vi "Trigger Sweep.vi"() -> ()   [LabVIEW 2011]
panel:
  out "Shots Measured":ext[][](array[numeric]) format="%#_10g"
  in  "Channel Delay (milliseconds)":u32=2500
  in  "Shot Delay (miliseconds)":u32
  in  "Shots":i32
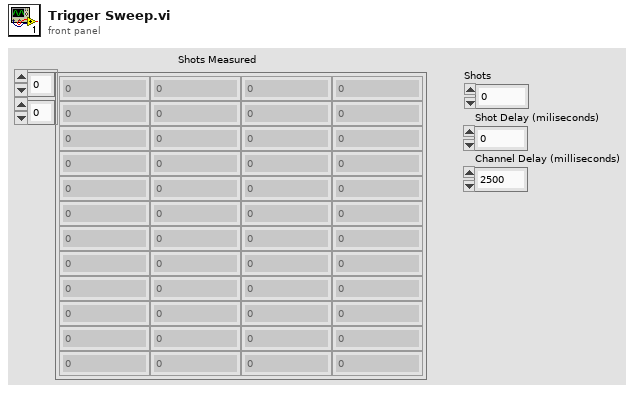
[diagram p1: front panel]
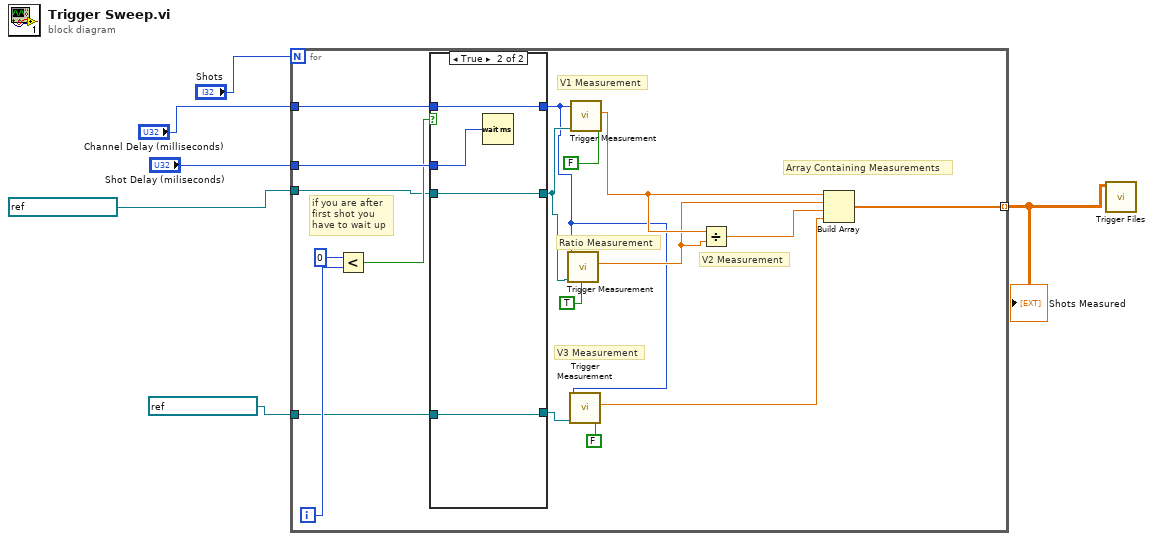
[diagram p0: block diagram]
diagram:
  n1 = for {
    N: "Shots" -> [_]
    tunnel: "Shot Delay (miliseconds)" -> [w24]
    tunnel: "Channel Delay (milliseconds)" -> [w20]
    tunnel: refnum<visa-resource-name> "GPIB0::7::INSTR" ("VISA resource name") -> [w19]
    tunnel: refnum<visa-resource-name> "GPIB0::5::INSTR" ("VISA resource name") -> [w11]
    tunnel: [w8] -> w1 mode=indexing
    i -> [w23]
    # "Array Containing Measurements"
    # "V3 Measurement"
    # "V2 Measurement"
    # "Ratio Measurement"
    # "V1 Measurement"
    # "if you are after\nfirst shot you\nhave to wait up"
    n2 = Less?(x=0, y=w23) -> (x < y?=w21:bool)
    n3 = case shown="True" w21 {
      tunnel: w24 -> [_ w31]
      tunnel: w20 -> [w27 w30]
      tunnel: [w27 w30] -> w7
      tunnel: w19 -> [w26 w29]
      tunnel: [w26 w29] -> w17
      tunnel: w11 -> [w25 w28]
      tunnel: [w25 w28] -> w10
      frame False {
      }
      frame True {
        n4 = Wait (ms)(milliseconds to wait=w31) -> ()  [unwired: 1 out]
      }
    }
    n5 = call "Trigger Measurement.vi"("Ratio Two Channels \n(Enable V1/V2 Measure)"=TRUE ("Ratio Two Channels \n(Enable V1/V2 Measure)"), "VISA resource name"=w17, "milliseconds to wait"=w7) -> ("Mean"=w14:dbl)  [unwired: 6 in, 2 out]
    n6 = call "Trigger Measurement.vi"("Ratio Two Channels \n(Enable V1/V2 Measure)"=FALSE ("Ratio Two Channels \n(Enable V1/V2 Measure)"), "VISA resource name"=w10, "milliseconds to wait"=w7) -> ("Mean"=w9:dbl)  [unwired: 6 in, 2 out]
    n7 = call "Trigger Measurement.vi"("Ratio Two Channels \n(Enable V1/V2 Measure)"=FALSE ("Ratio Two Channels \n(Enable V1/V2 Measure)"), "VISA resource name"=w17, "milliseconds to wait"=w7) -> ("Mean"=w15:dbl)  [unwired: 6 in, 2 out]
    n8 = Divide(x=w15, y=w14) -> (x/y=w13:dbl)
    n9 = Build Array(w15, w14, w13, w9) -> (w8:dbl[])
  }
  "Shots Measured" <- w1
  n10 = call "Trigger Files.vi"("2D data"=w1) -> ()  [unwired: 11 in]
